vi "Build Context Menu.vi"(8 "error in (no error)":errorcluster, 10 "MenuRef":refnum<k9>, 11 "HIJ Vision File Viewer in":refnum<class "HIJ Vision File Display.lvclass">) -> (0 "error out":errorcluster, 2 "MenuRef out":refnum<k9>, 3 "HIJ Vision File Viewer out":refnum<class "HIJ Vision File Display.lvclass">)   [LabVIEW 2014, in "HIJ Vision File Display.lvlib" / "HIJ Vision File Display.lvclass"]
uses:
  HIJ Vision File Display.lvclass
  Display Actors/HIJ Vision Display/HIJ Vision Display/HIJ Vision Display.lvclass
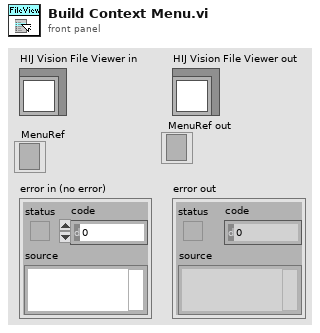
[diagram p1: front panel]
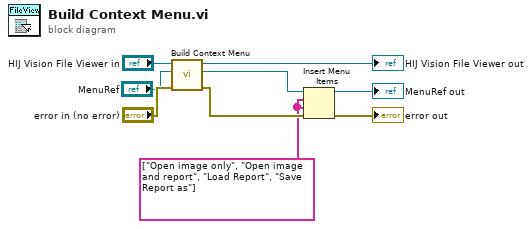
[diagram p0: block diagram]
diagram:
  w3 = string[] ["Open image only", "Open image and report", "Load Report", "Save Report as"] ("item names")
  n1 = call-parent "Build Context Menu.vi"("error in (no error)"="error in (no error)", "MenuRef"="MenuRef", "HIJ Vision Display in"="HIJ Vision File Viewer in") -> ("error out"=w5:errorcluster, "MenuRef out"=w2:refnum<k9>, "HIJ Vision Display out"=→"HIJ Vision File Viewer out":refnum<class "HIJ Vision File Display.lvclass">)  [unwired: 6 in]
  n2 = Insert Menu Items(6:w5, 7:w3, 8:w3, 9:w2) -> (0:→"error out":errorcluster, 3:→"MenuRef out":refnum<k9>)  [unwired: 2 in, 1 out]
